vi "ThingworxDemo.vi"() -> ()   [LabVIEW 2020]
uses:
  _TW_Subs/TW_XControl.xctl
  _TW_Subs/Thingworx_Write_Bool.vi
panel:
  in  "Boolean":bool
  in  "TW_XControl 2":string(xcontrol)
  out "number 2":dbl
  out "number":dbl
  in  "TW_XControl":string(xcontrol)
  # "Look at the diagram for more information"
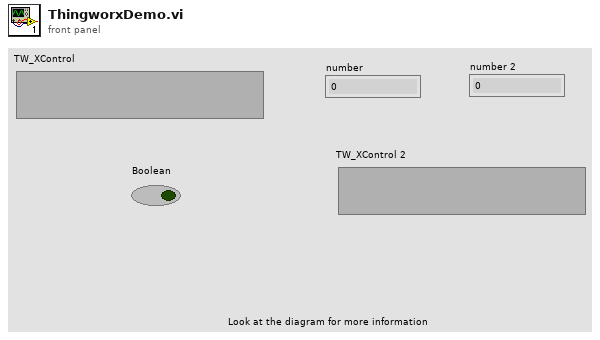
[diagram p1: front panel]
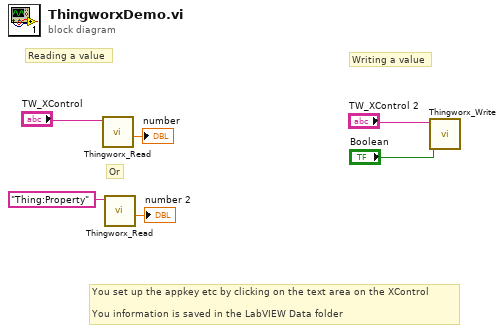
[diagram p0: block diagram]
diagram:
  # "You set up the appkey etc by clicking on the text area on the XControl\n\nYou information is saved in the LabVIEW Data folder"
  # "Writing a value"
  # "Reading a value"
  # "Or"
  n1 = call "Thingworx_Read.vi"("Thingworx"="TW_XControl") -> ("number"=→"number":dbl)  [unwired: 9 in, 1 out]
  n2 = call "Thingworx_Read.vi"("Thingworx"="Thing:Property") -> ("number"=→"number 2":dbl)  [unwired: 9 in, 1 out]
  n3 = call-poly "Thingworx_Write.vi"("Boolean"="Boolean", "Thingworx"="TW_XControl 2") -> ()  [unwired: 10 in]
